vi "Scheduler.Launch.vi"(8 "Error In":errorcluster, 11 "Q In":refnum<queue>) -> (0 "Error Out":errorcluster, 2 "Name":string, 3 "VI Refnum":refnum<vi>)   [LabVIEW 2024, in "EQMF.lvlib" / "Scheduler.lvlib"]
uses:
  Scheduler.lvlib
  Queues/Q.Element.ctl
  _Core/Scheduler.Service.vi
  Queues/Queue Utils.lvlib
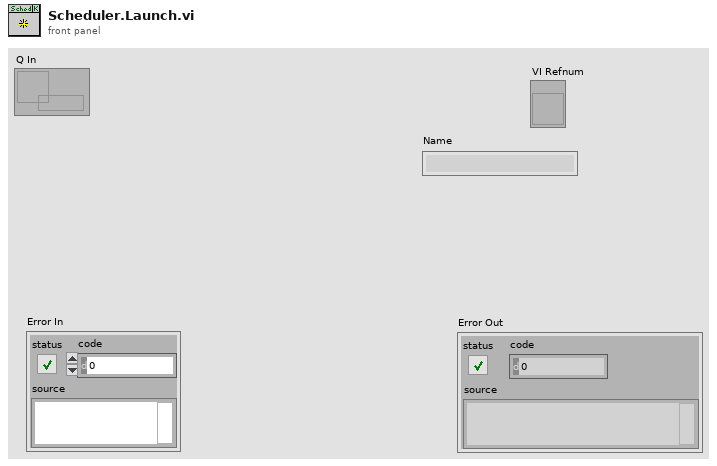
[diagram p1: front panel]
types:
  T1 = typedef "EQMF.lvlib/Queue Utils.lvlib/Q.Element.ctl" = cluster{"Cmd":string, "Sub":string, "Data1":variant, "Data2":variant}
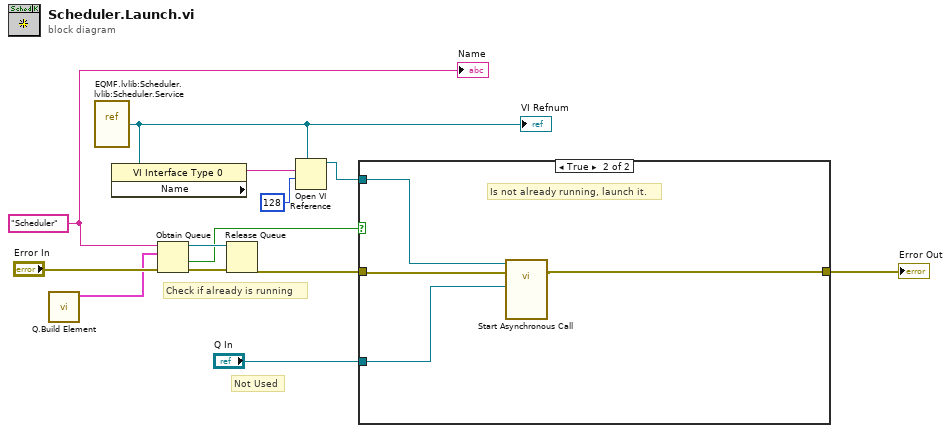
[diagram p0: block diagram]
diagram:
  w6 = "Scheduler" ("name (unnamed)")
  # "Not Used"
  # "Check if already is running"
  n1 = call "Q.Build Element.vi"() -> ("Q.Element"=w7:T1)  [unwired: 11 in]
  n2 = vi-ref "EQMF.lvlib:Scheduler.lvlib:Scheduler.Service.vi"() -> (w1:refnum<vi>)
  "VI Refnum" <- w1
  n3 = property class="VI Interface Type 0"(reference=w1) -> ("Name"=w4:string)  [unwired: 1 in, 2 out]
  n4 = Obtain Queue(name (unnamed)=w6, element data type=w7, error in (no error)="Error In") -> (queue out=w12:refnum<queue>, created new?=w8:bool, error out=w13:errorcluster)  [unwired: 2 in]
  n5 = Release Queue(queue=w12, error in (no error)=w13) -> (error out=w9:errorcluster)  [unwired: 1 in, 2 out]
  n6 = Open VI Reference(type specifier VI Refnum (for type only)=w1, vi path=w4, options=128) -> (vi reference=w2:refnum<vi>)  [unwired: 3 in, 1 out]
  n7 = case shown="True" w8 {
    tunnel: [w14 w17] -> w11
    tunnel: w9 -> [w14 w18]
    tunnel: "Q In" -> [_ w15]
    tunnel: w2 -> [_ w16]
    frame False {
      # "Is already running, do nothing"
    }
    frame True {
      # "Is not already running, launch it."
      n8 = call-by-ref "Start Asynchronous Call"(reference=w16, error in=w18, "Parent Q"=w15) -> (error out=w17:errorcluster)  [unwired: 11 in, 1 out]
    }
  }
  "Error Out" <- w11
  "Name" <- w6
